vi "M straight front S1.vi"() -> ()   [LabVIEW 2017]
uses:
  <vilib>/Rock Robotics/WPI/Framework/Completion Status.ctl
  <vilib>/Rock Robotics/WPI/Framework/Completion Notifier.ctl
  <vilib>/Rock Robotics/WPI/Framework/Command Status Info.ctl
  Support Code/Starting Position.ctl
  Support Code/Extended Block Inputs.ctl
panel:
  in  "Block Inputs":T1
  in  "switch Target Height (in)":dbl
  out "Command Info Out":T2
  in  "Starting Position":T5=enum."Far Right"
  in  "Command Info In":T2
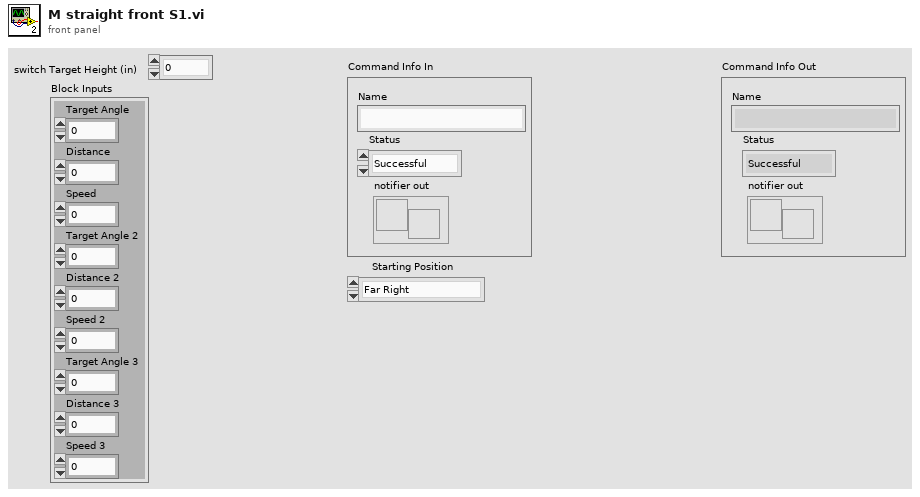
[diagram p1: front panel]
types:
  T1 = typedef "Extended Block Inputs.ctl" = cluster{"Target Angle":dbl, "Distance":dbl, "Speed":dbl, "Target Angle 2":dbl, "Distance 2":dbl, "Speed 2":dbl, "Target Angle 3":dbl, "Distance 3":dbl, "Speed 3":dbl}
  T2 = typedef "Command Status Info.ctl" = cluster{"Name":string, "Status":T3, "notifier out":T4}
  T3 = typedef "Completion Status.ctl" = enum16{"Successful", "Aborted", "Incomplete"}
  T4 = typedef "Completion Notifier.ctl" = refnum<notifier>
  T5 = typedef "Starting Position.ctl" = enum16{"Far Left", "Center", "Far Right"}
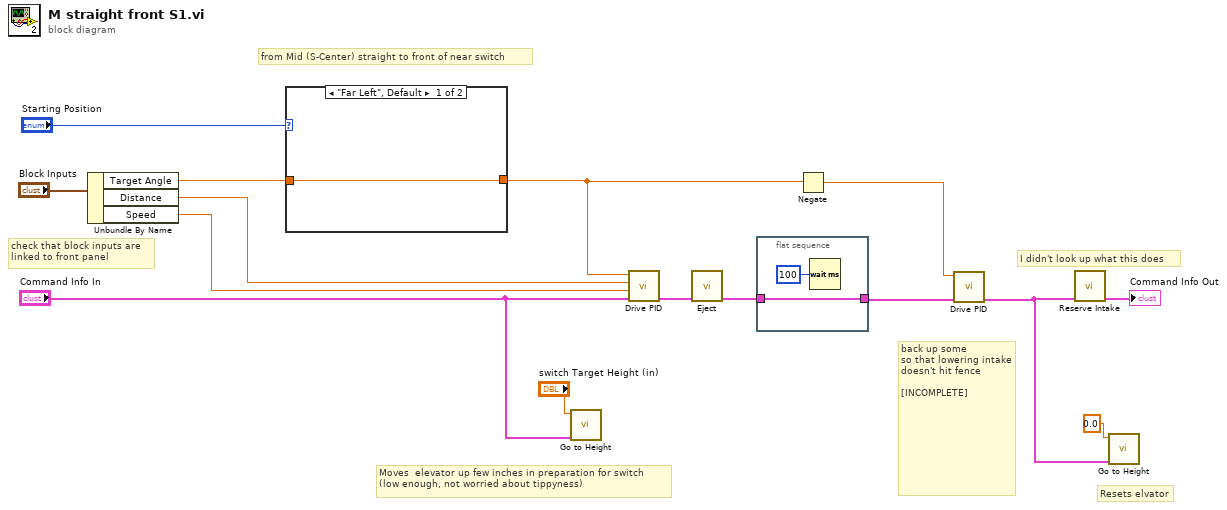
[diagram p0: block diagram]
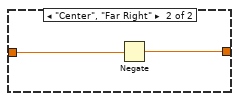
[diagram p2: hidden frame]
diagram:
  # "back up some\nso that lowering intake doesn't hit fence\n\n[INCOMPLETE]"
  # "I didn't look up what this does"
  # "Resets elvator"
  # "check that block inputs are\nlinked to front panel"
  # "Moves  elevator up few inches in preparation for switch\n(low enough, not worried about tippyness)"
  # "from Mid (S-Center) straight to front of near switch"
  n1 = Unbundle By Name("Block Inputs") -> ("Target Angle"=w10:dbl, "Distance"=w9:dbl, "Speed"=w8:dbl)
  n2 = case shown="\"Far Left\", Default" "Starting Position" {
    tunnel: [w16 w18] -> w2
    tunnel: w10 -> [w16 w17]
    frame "Far Left", Default {
    }
    frame "Center", "Far Right" {
      n3 = Negate(x=w17) -> (-x=w18:dbl)
    }
  }
  n4 = call "Go to Height.vi"("Command Info In"="Command Info In", "Target Height (in)"="switch Target Height (in)") -> ()  [unwired: 9 in, 1 out]
  n5 = call "Drive PID.vi"("Command Info In"="Command Info In", "Speed"=w8, "Distance"=w9, "Target Angle"=w2) -> ("Command Info Out"=w14:T2)  [unwired: 7 in]
  n6 = call "Eject.vi"("Command Info In"=w14) -> ("Command Info Out"=w13:T2)  [unwired: 10 in]
  n7 = flat-sequence {
    tunnel: w13 -> [w19]
    tunnel: [w19] -> w4
    frame #0 {
      n8 = Wait (ms)(milliseconds to wait=u32 100) -> ()  [unwired: 1 out]
    }
  }
  n9 = Negate(x=w2) -> (-x=w1:dbl)
  n10 = call "Drive PID.vi"("Command Info In"=w4, "Target Angle"=w1) -> ("Command Info Out"=w3:T2)  [unwired: 9 in]
  n11 = call "Reserve Intake.vi"("Command Info"=w3) -> ("Command Info"=→"Command Info Out":T2)  [unwired: 10 in]
  n12 = call "Go to Height.vi"("Command Info In"=w3, "Target Height (in)"=0.0) -> ()  [unwired: 9 in, 1 out]
